vi "Add VI to Library.vi"(8 "error in":errorcluster, 9 "VI":refnum<class "VI.lvclass">, 10 "VI Type":T1, 11 "Library in":refnum<class "Library.lvclass">) -> (0 "error out":errorcluster, 3 "Library out":refnum<class "Library.lvclass">)   [LabVIEW 2019, in "Panther Dashboard.lvlib" / "Library.lvclass"]
uses:
  Library.lvclass
  VI/VI.lvclass
  LabVIEWItem/Item Type--enum.ctl
  Library.lvclass/Library.ctl
  Read VIs MAP.vi
  Write VIs MAP.vi
  LabVIEWItem/LabVIEWItem.lvclass
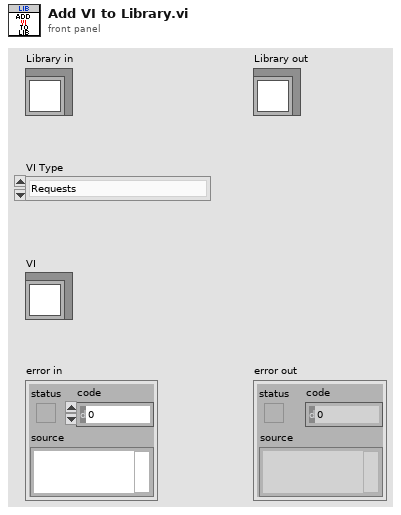
[diagram p1: front panel]
types:
  T1 = typedef "Panther Dashboard.lvlib/LabVIEWItem.lvclass/Item Type--enum.ctl" = enum16{"Requests", "Broadcasts", "Request and Wait for Reply", "Round Trip", "Public API VIs", "» Constant VIs", "» Error VIs", "Module", "Project"}
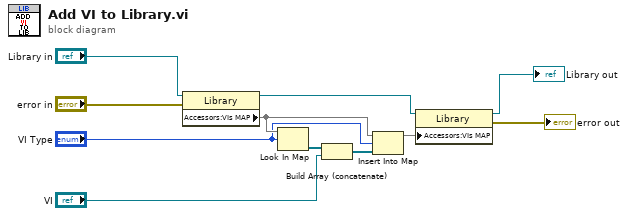
[diagram p0: block diagram]
diagram:
  n1 = property class="Library"(reference="Library in", error in="error in") -> (reference out=w9:refnum<class "Library.lvclass">, "Accessors:VIs MAP"=w5:map{T1, refnum<class "VI.lvclass">[]})  [unwired: 1 out]
  n2 = Look In Map(map=w5, key="VI Type") -> (value=w3:refnum<class "VI.lvclass">[])  [unwired: 1 in, 1 out]
  n3 = Build Array (concatenate)(w3, "VI") -> (w1:refnum<class "VI.lvclass">[])
  n4 = Insert Into Map(map in=w5, key="VI Type", value=w1) -> (map out=w6:map{T1, refnum<class "VI.lvclass">[]})  [unwired: 2 out]
  n5 = property class="Library"(reference=w9, "Accessors:VIs MAP"=w6) -> (reference out=→"Library out":refnum<class "Library.lvclass">, error out=→"error out":errorcluster)  [unwired: 1 in]
